vi "TCP Read.vi"(8 "error in (no error)":errorcluster, 9 "timeout":i32, 10 "bytes to read":i32, 11 "connection ID":refnum<k5>) -> (0 "error out":errorcluster, 1 "timed out?":bool, 2 "data":u8[](array[numeric]))   [LabVIEW 2018, in "SubVIs.lvlib" / "TCP Shared Components.lvlib"]
doc: "This function reads a TCP packet from the bus and checks for errors. It is a wrapper for standard functionality."
uses:
  TCP Shared Components.lvlib
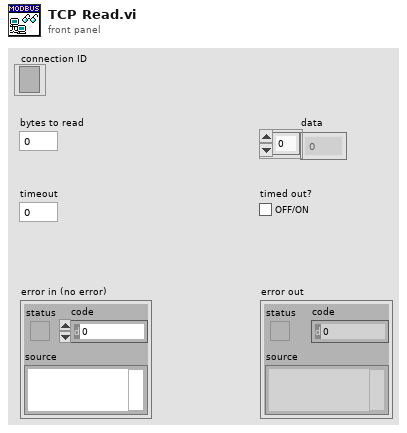
[diagram p1: front panel]
types:
  T1 = enum16{"Standard", "Buffered", "CRLF", "Immediate"}
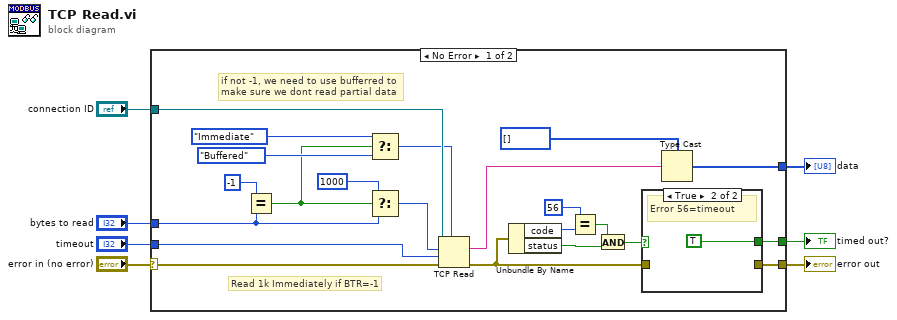
[diagram p0: block diagram]
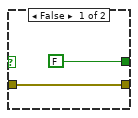
[diagram p2: hidden frame]
diagram:
  n1 = case shown="No Error" "error in (no error)" {
    selector: "error in (no error)" -> [w15 w33]
    tunnel: [w29 w33] -> w7
    tunnel: "timeout" -> [w28 _]
    tunnel: [w27 _] -> w5
    tunnel: "connection ID" -> [w26 _]
    tunnel: "bytes to read" -> [w18 _]
    tunnel: [w14 _] -> w1
    frame No Error {
      # "Read 1k Immediately if BTR=-1"
      # "if not -1, we need to use bufferred to\nmake sure we dont read partial data"
      n2 = Equal?(x=-1, y=w18) -> (x = y?=w19:bool)
      n3 = Select(t=T1."Immediate" ("mode (standard)"), s=w19, f=T1."Buffered" ("mode (standard)")) -> (s? t:f=w20:T1)
      n4 = Select(t=1000, s=w19, f=w18) -> (s? t:f=w17:i32)
      n5 = TCP Read(connection ID=w26, bytes to read=w17, error in (no error)=w15, 7:w20, 9:w28) -> (data out=w24:string, error out=w8:errorcluster)  [unwired: 1 out]
      n6 = Unbundle By Name(w8) -> ("code"=w13:i32, "status"=w10:bool)
      n7 = Equal?(x=56, y=w13) -> (x = y?=w11:bool)
      n8 = And(x=w11, y=w10) -> (x .and. y?=w9:bool)
      n9 = case shown="True" w9 {
        tunnel: w8 -> [w31 _]
        tunnel: [w31 _] -> w29
        tunnel: [FALSE TRUE] -> w14
        frame False {
        }
        frame True {
          # "Error 56=timeout"
        }
      }
      n10 = Type Cast(type=u8[] [] ("data"), x=w24) -> (*(type *) &x=w27:u8[])
    }
    frame Error {
    }
  }
  "error out" <- w7
  "data" <- w5
  "timed out?" <- w1
